vi "Present.vi"(8 "Stats":T1={"Transform And Project Duration"=0.0, "Raster Duration"=0.0, "Present Duration"=82.5692473, "Frame Rate"=111.70812900055276, "Visible Triangles"=0, "Delta Time"=0.0} {"Delta Time" format="%.0p"; "Frame Rate" format="%.0p"; "Present Duration" format="%.0p"; "Raster Duration" format="%.0p"; "Transform And Project Duration" format="%.0p"}, 9 "Display Stats":bool, 10 "Display Help":bool, 11 "Pixel Data":u32[][](array[numeric])) -> (2 "Present Duration [s]":dbl format="%.3p", 3 "2D Picture":picture)   [LabVIEW 2020, in "Example 1.lvlib"]
uses:
  Example 1.lvlib
  Graphics/Libraries/Utility/Utility.lvlib
  5bb89e80-4431-4a04-aab7-f6923ae8e18e.vi
  5002ab1c-b7b6-4038-93be-709e90c08d53.vi
  Scene/Stats.ctl
  Scene/Scene.lvclass
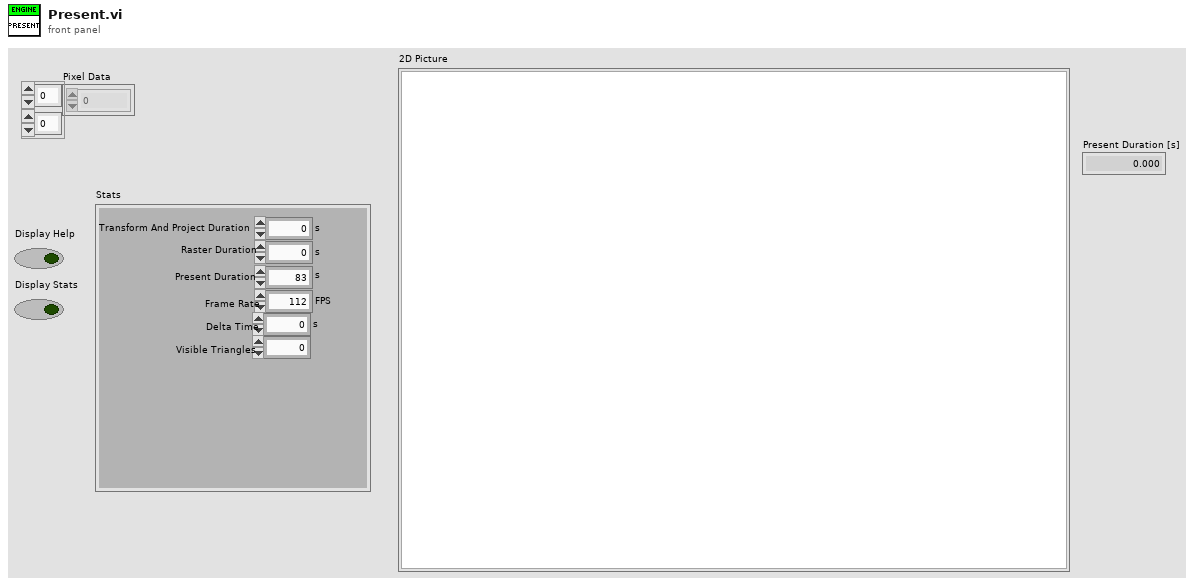
[diagram p1: front panel]
types:
  T1 = typedef "Scene.lvclass/Stats.ctl" = cluster{"Transform And Project Duration":dbl, "Raster Duration":dbl, "Present Duration":dbl, "Frame Rate":dbl, "Visible Triangles":i32, "Delta Time":dbl}
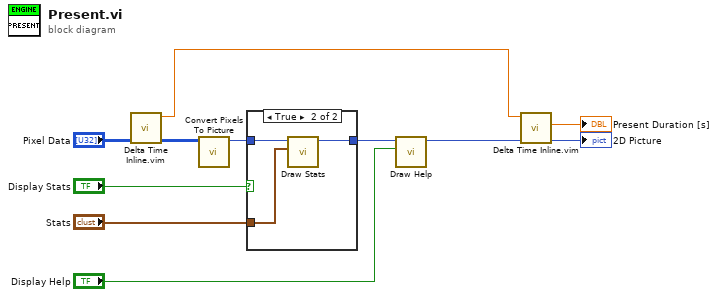
[diagram p0: block diagram]
diagram:
  n1 = call "Delta Time Inline.vim"("value in"="Pixel Data") -> ("value out"=w11:u32[][], "Relative Seconds out [s]"=w5:dbl)  [unwired: 8 in, 1 out]
  n2 = call "Convert Pixels To Picture.vi"("Pixel Data in"=w11) -> ("2D Picture"=w4:picture)  [unwired: 9 in, 1 out]
  n3 = case shown="True" "Display Stats" {
    tunnel: "Stats" -> [_ w15]
    tunnel: w4 -> [w12 w14]
    tunnel: [w12 w13] -> w2
    frame False {
    }
    frame True {
      n4 = call "Draw Stats.vi"("Stats"=w15, "Screen in"=w14) -> ("Screen out"=w13:picture)  [unwired: 9 in]
    }
  }
  n5 = call "Draw Help.vi"("Display Help"="Display Help", "Screen in"=w2) -> ("Screen out"=w7:picture)  [unwired: 9 in]
  n6 = call "Delta Time Inline.vim"("value in"=w7, "Relative Seconds in [s]"=w5) -> ("value out"=→"2D Picture":picture, "Delta Time [s]"=→"Present Duration [s]":dbl)  [unwired: 7 in, 1 out]
